vi "g_send.vi"(8 "error in (no error)":errorcluster, 10 "Input buffer size":u32=16384, 11 "USB Interface Name":refnum<visa-resource-name>="COM3") -> (0 "error out":errorcluster)   [LabVIEW 2012]
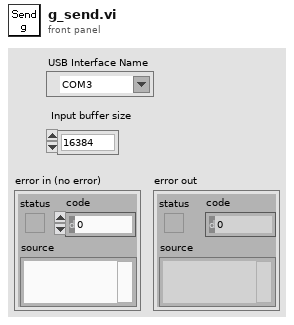
[diagram p1: front panel]
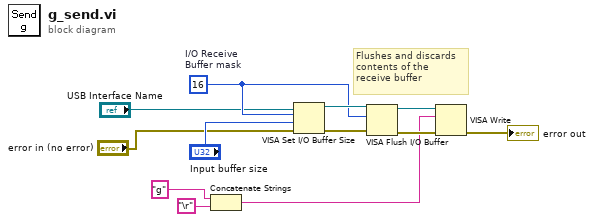
[diagram p0: block diagram]
diagram:
  w8 = u16 16  # I/O Receive Buffer mask
  # "Flushes and discards \ncontents of the \nreceive buffer"
  n1 = Concatenate Strings("g" ("Char to send"), "\r") -> (w3:string)
  n2 = VISA Set I/O Buffer Size(VISA resource name="USB Interface Name", mask (16)=w8, size (4096)="Input buffer size", error in (no error)="error in (no error)") -> (VISA resource name out=w10:refnum<visa-resource-name>, error out=w9:errorcluster)
  n3 = VISA Flush I/O Buffer(VISA resource name=w10, mask (16)=w8, error in (no error)=w9) -> (VISA resource name out=w12:refnum<visa-resource-name>, error out=w11:errorcluster)
  n4 = VISA Write(VISA resource name=w12, write buffer=w3, error in (no error)=w11) -> (error out=→"error out":errorcluster)  [unwired: 2 out]
